vi "Run_try1.vi"(7 "Team Index":i32, 8 "Column":i32, 9 "Row":i32, 10 "View":i32[](array[numeric]) caption="View (Team Index, -1: empty)", 11 "Atom In":refnum<class "Atom.lvclass">) -> (0 "Replicated":refnum<class "Square.lvclass">, 1 "Direction":T1=enum."E", 2 "Action":T2, 3 "Square Out":refnum<class "Square.lvclass">)   [LabVIEW 2017, in "Atom.lvclass"]
uses:
  Atom.lvclass
  C:/Users/Marty/Documents/squarebattle/Square/Square.lvclass
  Square/Square.lvclass
  Type Defs/Action Enum.ctl
  Type Defs/Direction Enum.ctl
  Atom.lvclass/Atom.ctl
  50f3e8b4-9c35-4f6c-8044-610a9d5e60e8.vi
  Type Defs/SB Type Defs.lvlib
panel:
  # "NW\nN\nNE\nE\nSE\nS\nSW\nW"
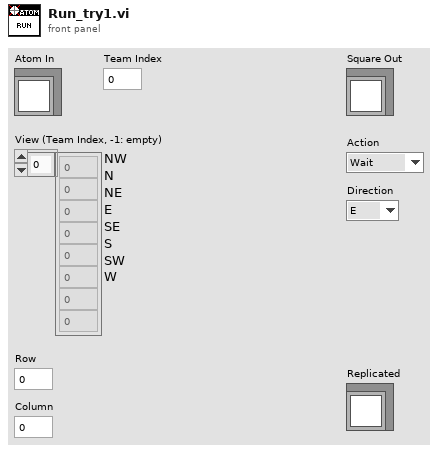
[diagram p1: front panel]
types:
  T1 = typedef "SB Type Defs.lvlib/Direction Enum.ctl" = enum16{"NW", "N", "NE", "E", "SE", "S", "SW", "W"}
  T2 = typedef "SB Type Defs.lvlib/Action Enum.ctl" = enum16{"Wait", "Move", "Attack", "Replicate"}
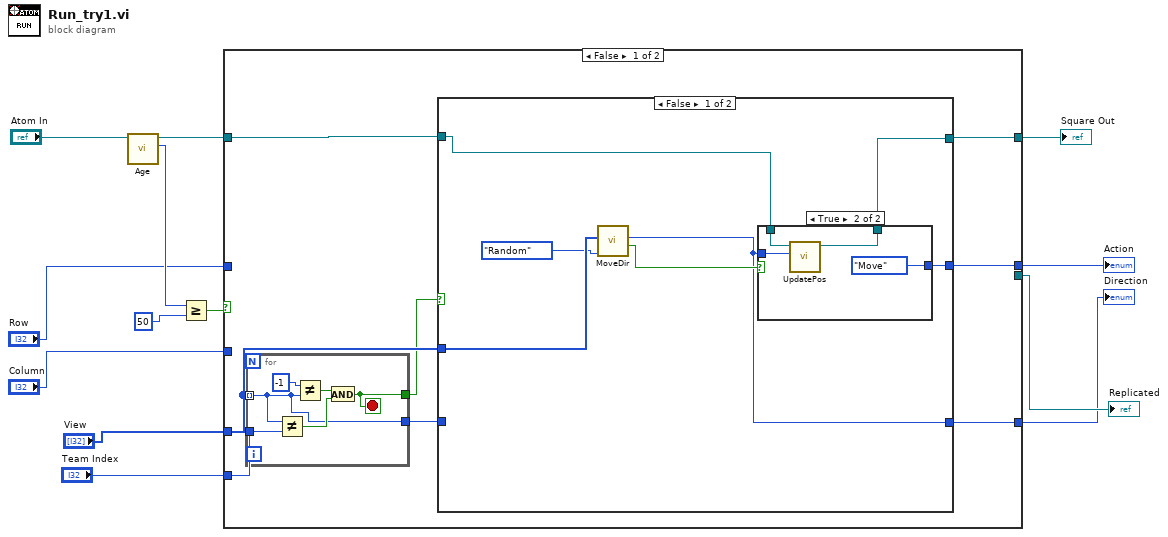
[diagram p0: block diagram]
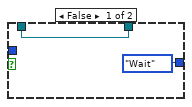
[diagram p2: hidden frame]
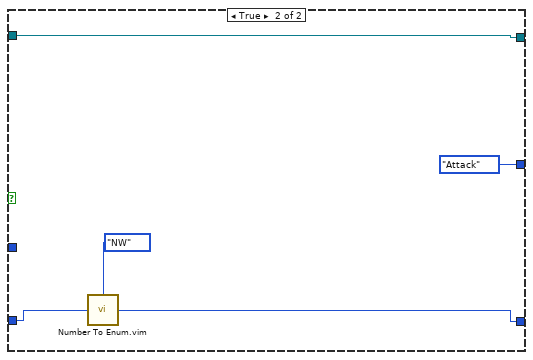
[diagram p3: hidden frame]
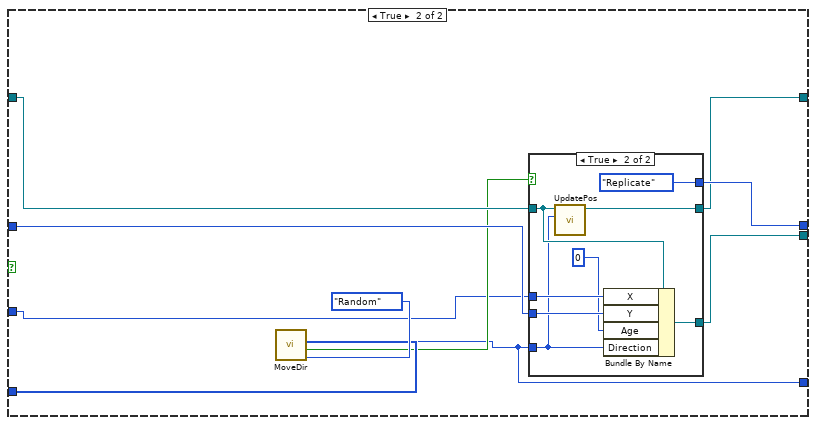
[diagram p4: hidden frame]
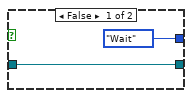
[diagram p5: hidden frame]
diagram:
  n1 = call "Age.vi"("Atom In"="Atom In") -> ("Current Age"=w8:i32, "Atom Out"=w6:refnum<class "Atom.lvclass">)  [unwired: 9 in]
  n2 = Greater Or Equal?(x=w8, y=50) -> (x >= y?=w1:bool)
  n3 = case shown="False" w1 {
    tunnel: [w20 w51] -> w13
    tunnel: w6 -> [w15 w52]
    tunnel: [w21 w55] -> w11
    tunnel: "View" -> [w18 w49]
    tunnel: "Team Index" -> [w19 _]
    tunnel: "Column" -> [_ w47]
    tunnel: "Row" -> [_ w54]
    tunnel: [_ w53] -> w3
    tunnel: [w14 w46] -> w2
    frame False {
      n4 = for {
        tunnel: w18 -> [w22] mode=indexing
        tunnel: w19 -> [w24]
        tunnel: [w23] -> w17
        tunnel: [w22] -> w16
        stop <- w23 stop-if-true
        n5 = Not Equal?(x=w22, y=w24) -> (x != y?=w25:bool)
        n6 = Not Equal?(x=-1, y=w22) -> (x != y?=w26:bool)
        n7 = And(x=w26, y=w25) -> (x .and. y?=w23:bool)
      }
      n8 = case shown="False" w17 {
        tunnel: [w34 Action_Enum."Attack" ("Action")] -> w21
        tunnel: [w33 w45] -> w20
        tunnel: w18 -> [w31 _]
        tunnel: w15 -> [w32 w45]
        tunnel: w16 -> [_ w42]
        tunnel: [w28 w41] -> w14
        frame False {
          n9 = call "MoveDir.vi"("Type"=enum16{"Random", "Simple"}."Random", "View"=w31) -> ("ValidDir"=w29:bool, "Direction"=w28:T1)  [unwired: 7 in, 1 out]
          n10 = case shown="True" w29 {
            tunnel: [Action_Enum."Wait" ("Action") Action_Enum."Move" ("Action")] -> w34
            tunnel: w32 -> [w35 w39]
            tunnel: [w35 w38] -> w33
            tunnel: w28 -> [_ w37]
            frame False {
            }
            frame True {
              n11 = call "UpdatePos.vi"("Direction"=w37, "Atom In"=w39) -> ("Atom Out"=w38:refnum<class "Atom.lvclass">)  [unwired: 9 in]
            }
          }
        }
        frame True {
          n12 = call "Number To Enum.vim"("number"=w42, "enum type"=Direction_Enum."NW" ("Direction")) -> ("number as enum"=w41:T1)
        }
      }
    }
    frame True {
      n13 = call "MoveDir.vi"("Type"=enum16{"Random", "Simple"}."Random", "View"=w49) -> ("ValidDir"=w48:bool, "Direction"=w46:T1)  [unwired: 7 in, 1 out]
      n14 = case shown="True" w48 {
        tunnel: [Action_Enum."Wait" ("Action") Action_Enum."Replicate" ("Action")] -> w55
        tunnel: [w56 w64] -> w51
        tunnel: w52 -> [w56 w59]
        tunnel: w47 -> [_ w63]
        tunnel: w54 -> [_ w62]
        tunnel: [_ w60] -> w53
        tunnel: w46 -> [_ w58]
        frame False {
        }
        frame True {
          n15 = call "UpdatePos.vi"("Direction"=w58, "Atom In"=w59) -> ("Atom Out"=w64:refnum<class "Atom.lvclass">)  [unwired: 9 in]
          n16 = Bundle By Name(cluster=w59, "X"=w63, "Y"=w62, "Age"=0, "Direction"=w58) -> (w60:refnum<class "Atom.lvclass">)
        }
      }
    }
  }
  "Square Out" <- w13
  "Action" <- w11
  "Direction" <- w2
  "Replicated" <- w3
